vi "Pre Launch Init.vi"(11 "Assert Startup UI in":refnum<class "Assert Startup UI.lvclass">) -> (0 "error out":errorcluster, 3 "Assert Startup UI out":refnum<class "Assert Startup UI.lvclass">)   [LabVIEW 2016, in "Assert Startup UI.lvlib" / "Assert Startup UI.lvclass"]
doc: "(<B>Filename</B>: Actor Framework.lvlib:Actor.lvclass:Pre Launch Init.vi)\n\nDefines behavior that occurs after the Launch Nested Actor method is invoked but before the actor's Actor Core method begins running.\n\nBy default, this method does nothing. A descendant class may override it to define behavior."
uses:
  Assert Startup UI.lvclass
  <vilib>/ActorFramework/Message Enqueuer/Message Enqueuer.lvclass
  Assert Startup UI.lvclass/Assert Startup UI.ctl
  Base UI Actor/Base UI Actor/Base UI Actor.lvclass
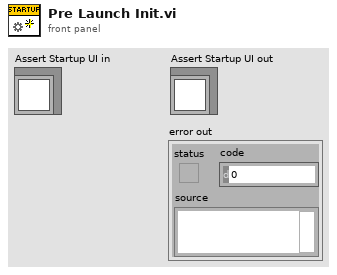
[diagram p1: front panel]
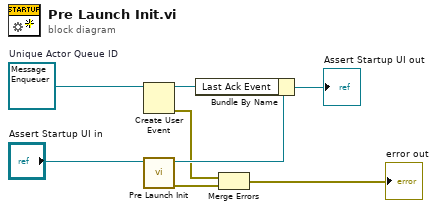
[diagram p0: block diagram]
diagram:
  w5 = refnum<class "Message Enqueuer.lvclass"> refnum  # Unique Actor Queue ID
  n1 = Create User Event(user event datatype=w5) -> (user event=w3:refnum<user-event>, error out=w1:errorcluster)  [unwired: 1 in]
  n2 = call-parent "Pre Launch Init.vi"("Base UI Actor in"="Assert Startup UI in") -> ("error out"=w8:errorcluster, "Base UI Actor out"=w7:refnum<class "Assert Startup UI.lvclass">)  [unwired: 9 in]
  n3 = Bundle By Name(cluster=w7, "Last Ack Event"=w3) -> (→"Assert Startup UI out":refnum<class "Assert Startup UI.lvclass">)
  n4 = Merge Errors(w1, w8) -> (→"error out":errorcluster)
